vi "Read Last of Header Contents Class Array.vi"(8 "error in (no error)":errorcluster, 11 "Save Image in":refnum<class "Save Image.lvclass">) -> (0 "error out":errorcluster, 2 "Simulated_Header.lvclass":refnum<class "Simulated_Header.lvclass">, 3 "Save Image out":refnum<class "Save Image.lvclass">)   [LabVIEW 2018, in "Save Image.lvclass"]
uses:
  Save Image.lvclass
  Simulated_Header/Simulated_Header.lvclass
  Save Image.lvclass/Save Image.ctl
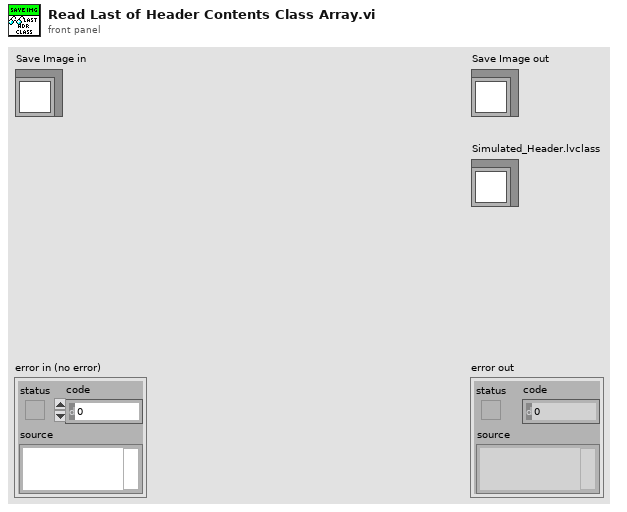
[diagram p1: front panel]
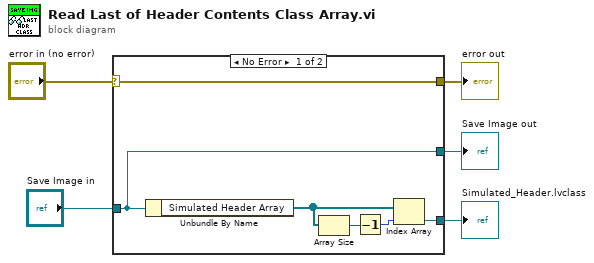
[diagram p0: block diagram]
diagram:
  n1 = case shown="No Error" "error in (no error)" {
    selector: "error in (no error)" -> [w11 w12]
    tunnel: [w11 w12] -> w4
    tunnel: [w10 w13] -> w2
    tunnel: "Save Image in" -> [w10 w13]
    tunnel: [w9 _] -> w1
    frame No Error {
      n2 = Unbundle By Name(w10) -> ("Simulated Header Array"=w8:refnum<class "Simulated_Header.lvclass">[])
      n3 = Array Size(array=w8) -> (size(s)=w7:i32)
      n4 = Decrement(x=w7) -> (x-1=w6:i32)
      n5 = Index Array(array=w8, index=w6) -> (element=w9:refnum<class "Simulated_Header.lvclass">)
    }
    frame Error {
    }
  }
  "error out" <- w4
  "Save Image out" <- w2
  "Simulated_Header.lvclass" <- w1
